vi "33333333333.vi"() -> ()   [LabVIEW 2017]
panel:
  in  ".bat":T1={"getVersion"="Getting Software Version.bat", "Start Test mode"="Start Test Mode.bat", "Start camera test mode"="Stop camera test mode.bat", "get one RAW Image"="Get one image.bat", "Stop camera test mode"="Stop camera test mode.bat", "Stop Test Mode"="Stop Test Mode.bat", "Get image reflection"="Get image reflection.bat", "Get image uniformity andFlash LED brightness"="Get image uniformity andFlash LED brightness.bat", "Disable flash LED"="Disable flash LED.bat", "Enable flash LED"="Enable flash LED.bat", "Software Reset"="Software Reset.bat", "Tune Flash LED brightness"="Tune Flash LED brightness.bat", "Start Camera calibration"="Start Camera calibration.bat", "TBD"="TBD.bat"}
  in  "base path":path
  in  "file path (use dialog)":path
  in  "错误输入（无错误）":errorcluster
  out "错误输出":errorcluster
  out "error  out":errorcluster
  in  "error in (no error)":errorcluster
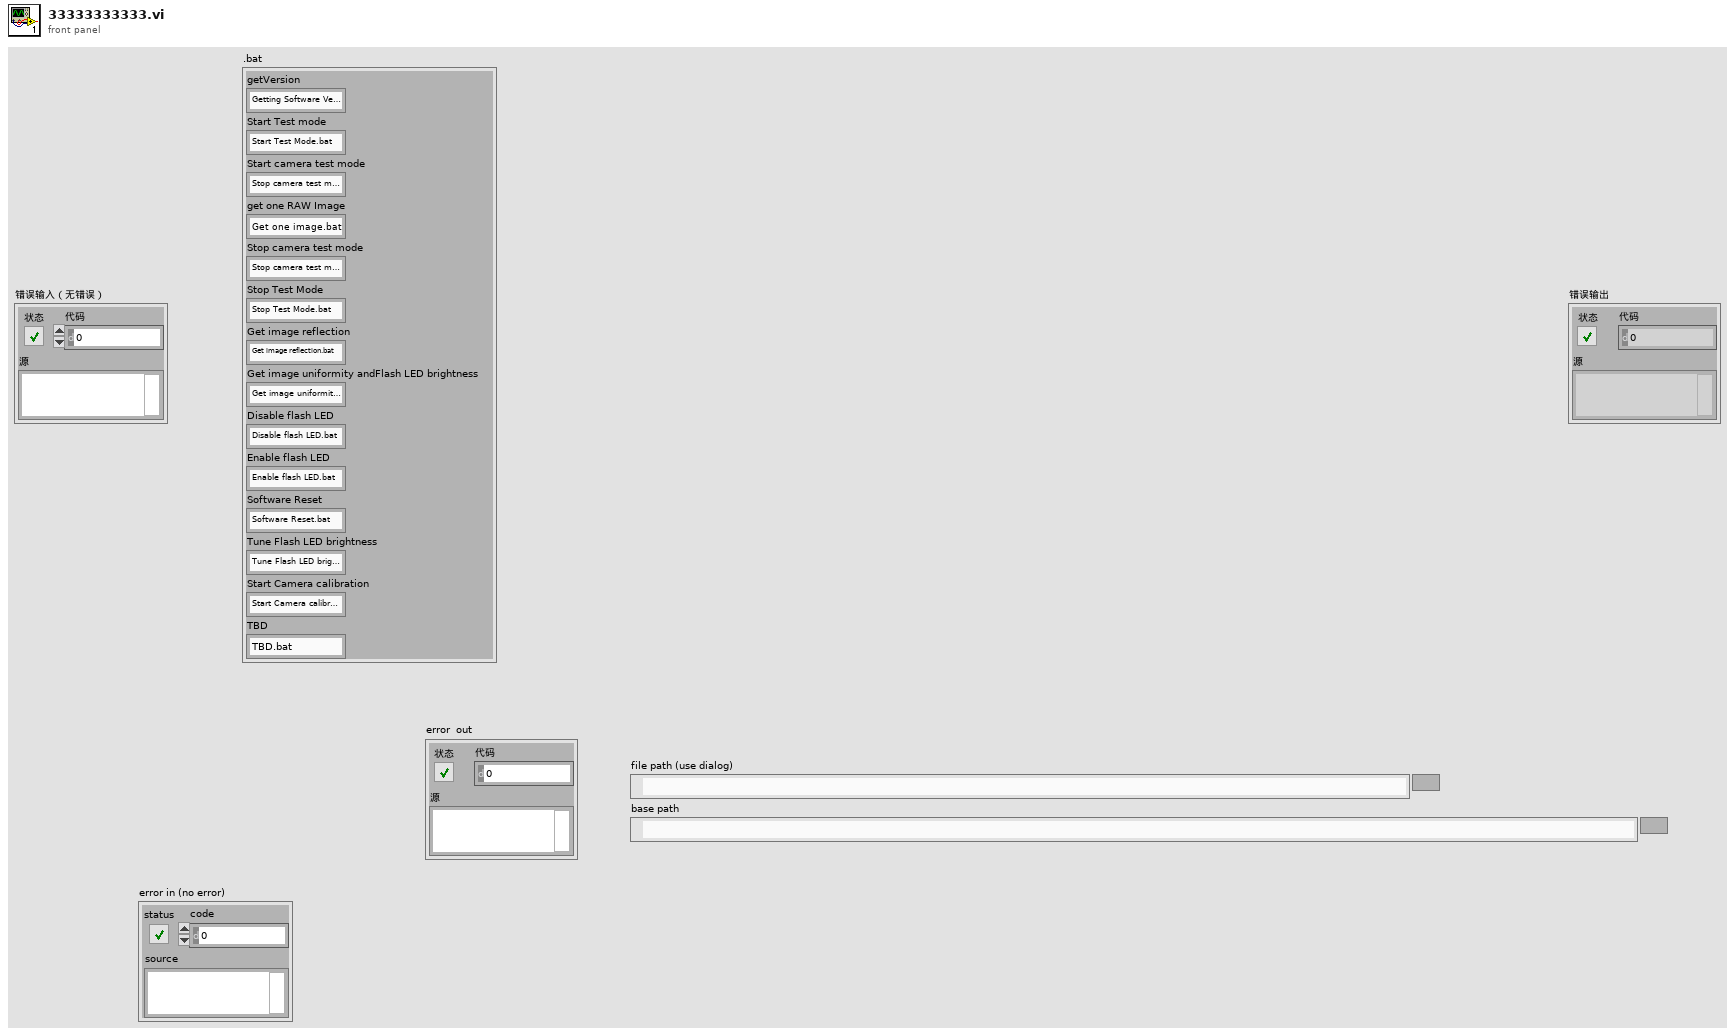
[diagram p1: front panel]
types:
  T1 = cluster{"getVersion":string, "Start Test mode":string, "Start camera test mode":string, "get one RAW Image":string, "Stop camera test mode":string, "Stop Test Mode":string, "Get image reflection":string, "Get image uniformity andFlash LED brightness":string, "Disable flash LED":string, "Enable flash LED":string, "Software Reset":string, "Tune Flash LED brightness":string, "Start Camera calibration":string, "TBD":string}
  T2 = enum16{"open", "replace", "create", "open or create", "replace or create", "replace or create with confirmation"}
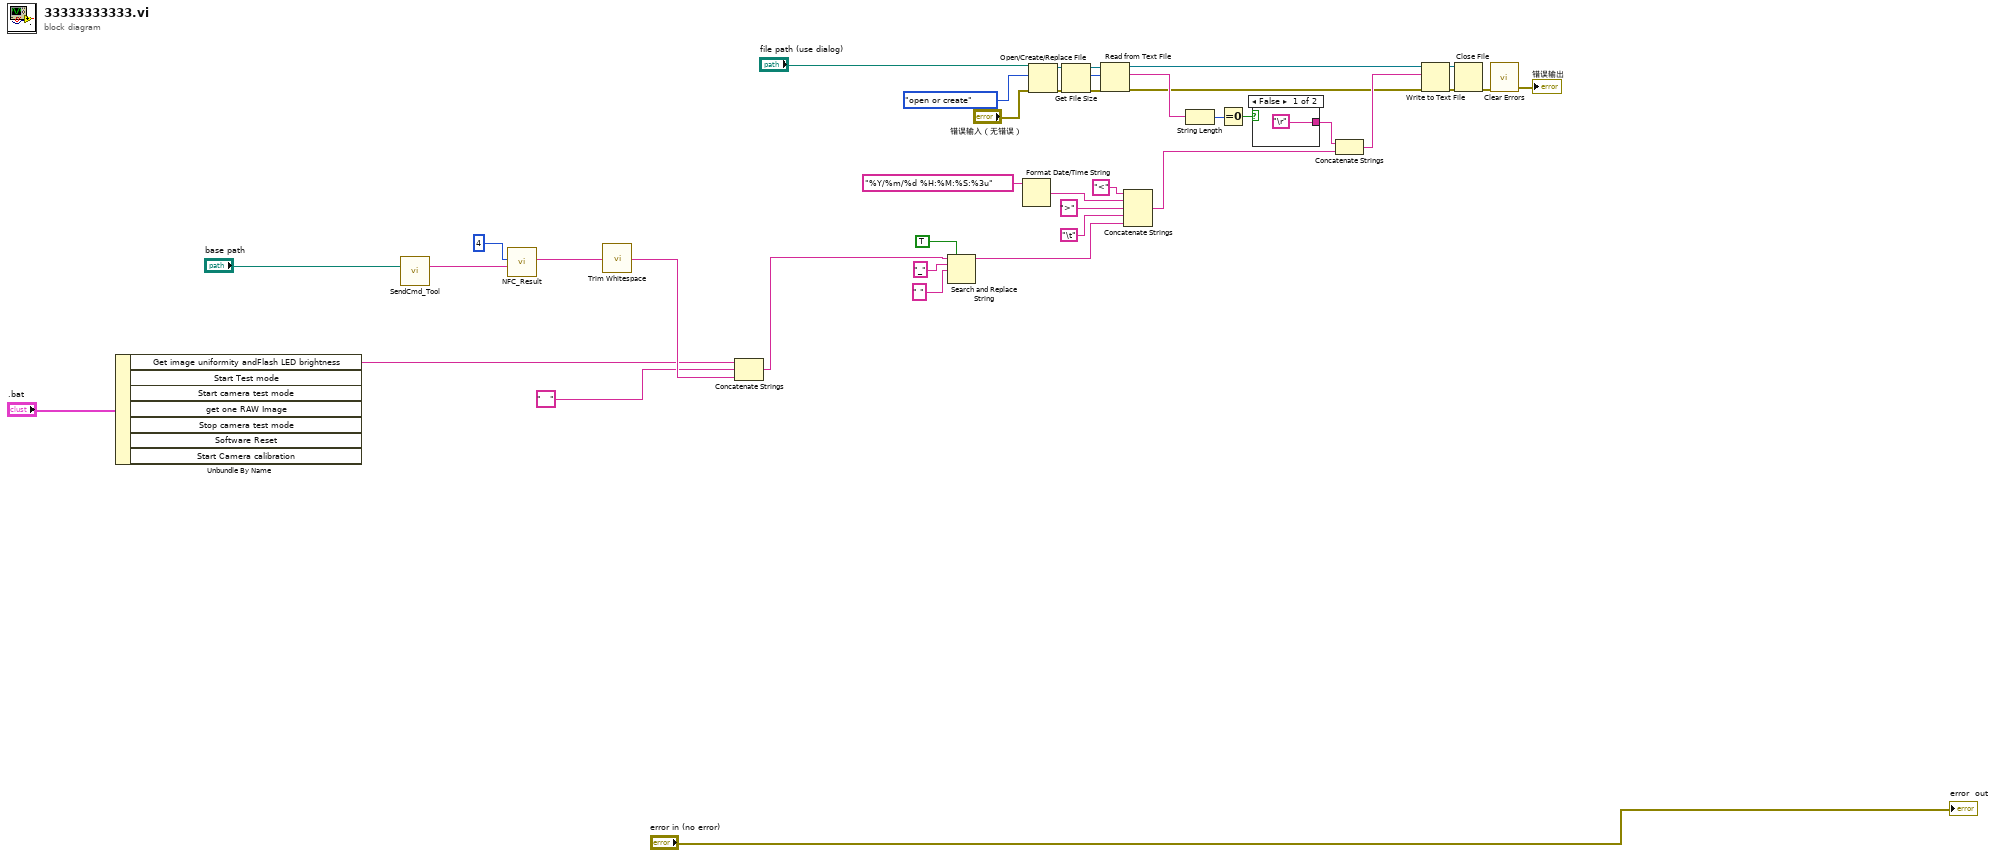
[diagram p0: block diagram]
diagram:
  n1 = Unbundle By Name(".bat") -> ("Get image uniformity andFlash LED brightness"=w1:string)  [unwired: 6 out]
  n2 = call "SendCmd_Tool.vi"("path_bat"="base path") -> ("Other"=w7:string)  [unwired: 9 in, 5 out]
  n3 = call "NFC_Result.vi"("input"=w7, "return code"=4) -> ("return_result"=w9:string)  [unwired: 8 in, 1 out]
  n4 = call <vilib>:"Trim Whitespace.vi"("string"=w9) -> ("trimmed string"=w4:string)  [unwired: 1 in]
  n5 = Concatenate Strings(w1, "   ", w4) -> (w5:string)
  n6 = Search and Replace String(replace all?=TRUE ("替换全部？(F)"), input string=w5, search string="_" ("搜索字符串"), replace string=" " ("替换字符串(\"\")")) -> (result string=w30:string)  [unwired: 4 in, 3 out]
  n7 = Format Date/Time String(time format string (%c)="%Y/%m/%d %H:%M:%S:%3u" ("时间格式字符串(%c)")) -> (date/time string=w35:string)  [unwired: 2 in]
  n8 = Open/Create/Replace File(file path (use dialog)="file path (use dialog)", error in="错误输入（无错误）", operation (0:open)=T2."open or create" ("操作(0:open)")) -> (refnum out=w13:refnum<file>, error out=w14:errorcluster)  [unwired: 3 in, 1 out]
  n9 = Get File Size ("获取文件大小")(file=w13, error in=w14) -> (refnum out=w15:refnum<file>, size (in bytes)=w17:i64, 0:w16:errorcluster)
  n10 = Read from Text File ("读取文本文件")(file (use dialog)=w15, count=w17, error in=w16) -> (refnum out=w18:refnum<file>, text=w22:string, error out=w19:errorcluster)  [unwired: 1 in, 1 out]
  n11 = Concatenate Strings("<" ("字符串"), w35, ">" ("字符串"), "\t", w30) -> (w11:string)
  n12 = String Length(string=w22) -> (length=w21:i32)
  n13 = Equal To 0?(x=w21) -> (x = 0?=w20:bool)
  n14 = case shown="False" w20 {
    tunnel: ["\r" _] -> w23
    frame False {
    }
    frame True {
    }
  }
  n15 = Concatenate Strings(w23, w11) -> (w24:string)
  n16 = Write to Text File ("写入文本文件")(file (use dialog)=w18, text=w24, error in=w19) -> (refnum out=w25:refnum<file>, error out=w26:errorcluster)  [unwired: 1 in, 1 out]
  n17 = Close File(refnum=w25, error in=w26) -> (error out=w28:errorcluster)  [unwired: 1 out]
  n18 = call <vilib>:"Clear Errors.vi"("error in (no error)"=w28) -> ("error out"=→"错误输出":errorcluster)  [unwired: 5 in, 1 out]
  "error  out" <- "error in (no error)"
